vi "From XML.vi"(8 "error in (no error)":errorcluster, 10 "XML String":string, 11 "Topic in":refnum<class "Topic.lvclass">) -> (0 "error out":errorcluster, 3 "Topic out":refnum<class "Topic.lvclass">)   [LabVIEW 2027, in "Topic.lvclass"]
uses:
  Topic.lvclass
  <vilib>/NI/Compiled HTML Menu Tool/Keyed Value Tree/Keyed Value Tree.lvclass
  Topic.lvclass/Topic.ctl
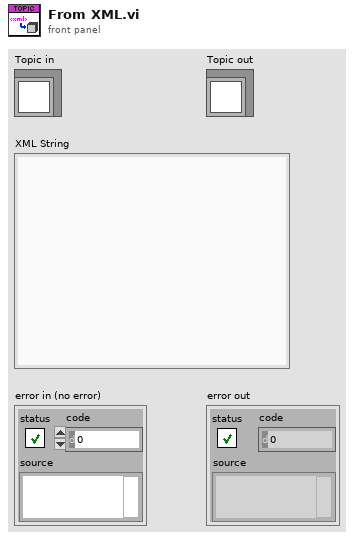
[diagram p1: front panel]
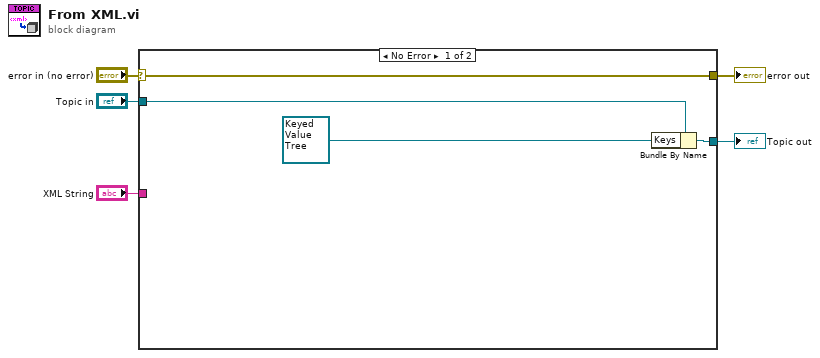
[diagram p0: block diagram]
diagram:
  n1 = case shown="No Error" "error in (no error)" {
    selector: "error in (no error)" -> [w9 w11]
    tunnel: [w9 w11] -> w4
    tunnel: [w6 w10] -> w2
    tunnel: "Topic in" -> [w7 w10]
    tunnel: "XML String" -> [_ _]
    frame No Error {
      n2 = Bundle By Name(cluster=w7, "Keys"=refnum<class "Keyed Value Tree.lvclass"> refnum ("Keyed Value Tree.lvclass")) -> (w6:refnum<class "Topic.lvclass">)
    }
    frame Error {
    }
  }
  "error out" <- w4
  "Topic out" <- w2
